vi "destroy_lookup.vi"(8 "error in (no error)":errorcluster, 11 "Mapped Lookup in":refnum<class "Mapped Lookup.lvclass">) -> (0 "error out":errorcluster, 1 "remaining references":refnum<data-value>[](array[refnum]))   [LabVIEW 2019, in "Lookup API.lvlib" / "Mapped Lookup.lvclass"]
uses:
  Mapped Lookup.lvclass
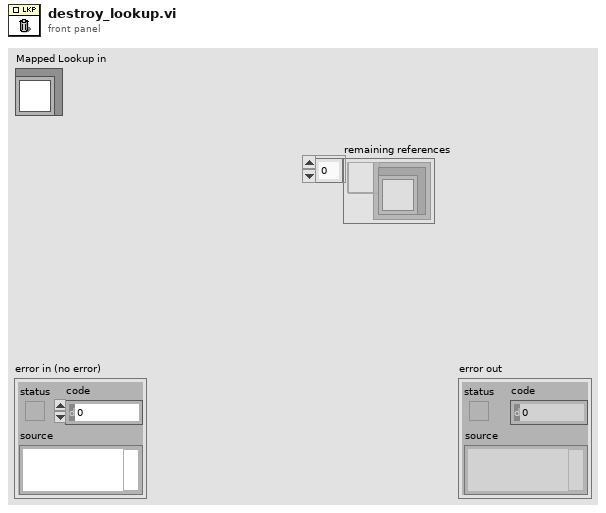
[diagram p1: front panel]
types:
  T1 = map{string, cluster{"instances":refnum<data-value>, "events":refnum<data-value>}}
  T2 = cluster{"instances":refnum<data-value>, "events":refnum<data-value>}
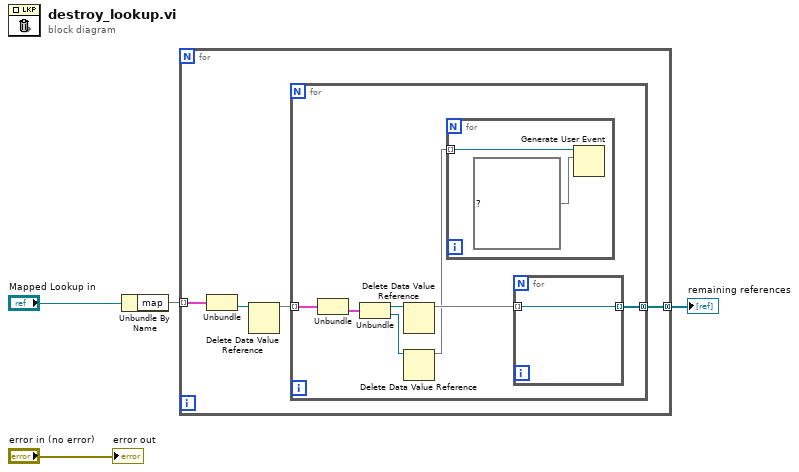
[diagram p0: block diagram]
diagram:
  n1 = Unbundle By Name("Mapped Lookup in") -> ("map"=w3:map{refnum<class>, refnum<data-value>})
  n2 = for {
    tunnel: w3 -> [w8] mode=indexing
    tunnel: [w5] -> w1 mode=concatenating
    n3 = Unbundle(w8) -> ("named instances"=w7:refnum<data-value>)  [unwired: 1 out]
    n4 = Delete Data Value Reference(data value reference=w7) -> (data value=w6:T1)  [unwired: 1 in, 1 out]
    n5 = for {
      tunnel: w6 -> [w15] mode=indexing
      tunnel: [w9] -> w5 mode=concatenating
      n6 = Unbundle(w15) -> (w14:T2)  [unwired: 1 out]
      n7 = Unbundle(w14) -> ("instances"=w13:refnum<data-value>, "events"=w12:refnum<data-value>)
      n8 = Delete Data Value Reference(data value reference=w13) -> (data value=w11:set{refnum<data-value>})  [unwired: 1 in, 1 out]
      n9 = Delete Data Value Reference(data value reference=w12) -> (data value=w10:set{refnum<user-event>})  [unwired: 1 in, 1 out]
      n10 = for {
        tunnel: w10 -> [w17] mode=indexing
        n11 = Generate User Event(user event=w17, event data cluster=set{refnum<data-value>} {} ("event data")) -> ()  [unwired: 2 in, 2 out]
      }
      n12 = for {
        tunnel: w11 -> [w18] mode=indexing
        tunnel: [w18] -> w9 mode=indexing
      }
    }
  }
  "remaining references" <- w1
  "error out" <- "error in (no error)"
